vi "Update Subs.vi"(8 "error in":errorcluster, 9 "Sub-Ctl Ref":refnum<vi>, 10 "Sub Control":T1) -> (0 "error out":errorcluster)   [LabVIEW 2020, in "Navigation.lvlib" / "Button Manager.lvclass"]
doc: "____\nHAMPEL SOFTWARE ENGINEERING v2.6.0 (2023-12-19 10:54)"
uses:
  Button Manager.lvclass
  Sub Control.ctl
  <vilib>/Utility/error.llb/Error Cluster From Error Code.vi
  <vilib>/ErrorRing/Error Ring.xnode
  Button Manager.lvclass/Button Manager.ctl
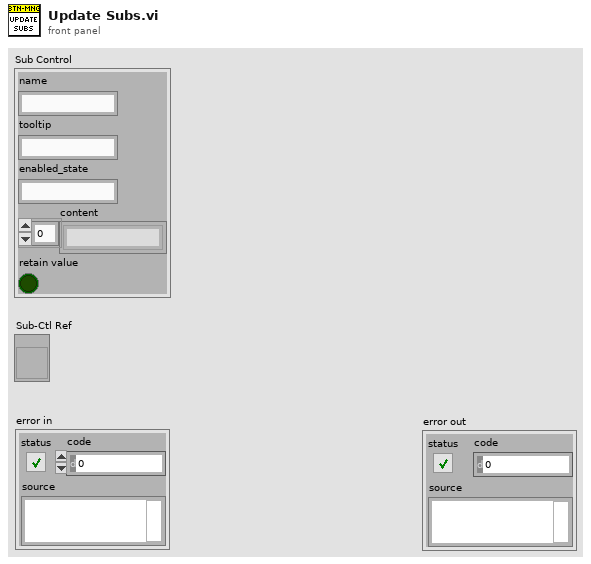
[diagram p1: front panel]
types:
  T1 = typedef "Navigation.lvlib/Button Manager.lvclass/Sub Control.ctl" = cluster{"name":string, "tooltip":string, "enabled_state":string, "content":string[], "retain value":bool}
  T2 = enum8{"Enabled", "Disabled", "Disabled and Grayed Out"}
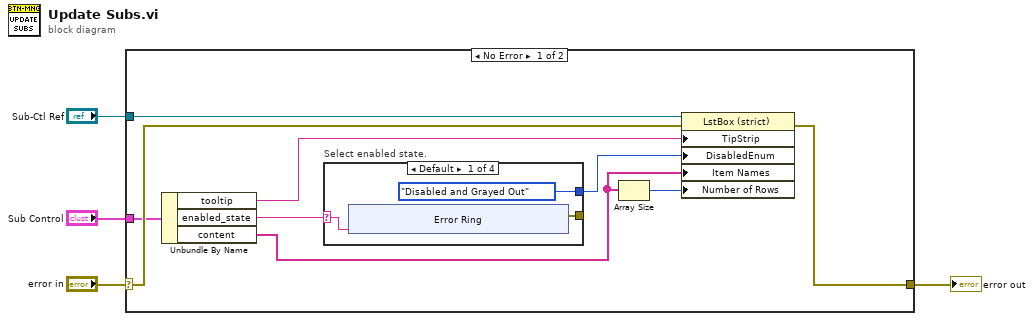
[diagram p0: block diagram]
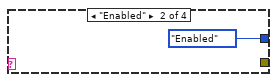
[diagram p2: hidden frame]
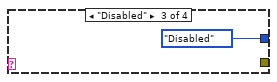
[diagram p3: hidden frame]
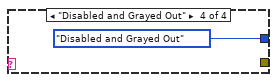
[diagram p4: hidden frame]
diagram:
  n1 = case shown="No Error" "error in" {
    selector: "error in" -> [w13 w27]
    tunnel: [w5 w27] -> w3
    tunnel: "Sub Control" -> [w12 _]
    tunnel: "Sub-Ctl Ref" -> [w11 _]
    frame No Error {
      n2 = Unbundle By Name(w12) -> ("tooltip"=w10:string, "enabled_state"=w9:string, "content"=w7:string[])
      n3 = case "Select enabled state." shown="Default" w9 {
        selector: w9 -> [w15 _ _ _]
        tunnel: [T2."Disabled and Grayed Out" ("Disabled") T2."Enabled" ("Disabled") T2."Disabled" ("Disabled") T2."Disabled and Grayed Out" ("Disabled")] -> w8
        tunnel: [w14 _ _ _] -> _
        frame Default {
          n4 = xnode "Error Ring"("parameter 0"=w15) -> ("error out"=w14:errorcluster)
        }
        frame "Enabled" {
        }
        frame "Disabled" {
        }
        frame "Disabled and Grayed Out" {
        }
      }
      n5 = Array Size(array=w7) -> (size(s)=w6:i32)
      n6 = property class="LstBox (strict)"(reference=w11, error in=w13, "TipStrip"=w10, "DisabledEnum"=w8, "Item Names"=w7, "Number of Rows"=w6) -> (error out=w5:errorcluster)  [unwired: 1 out]
    }
    frame Error {
    }
  }
  "error out" <- w3
